vi "hold_queues_in_memory.vi"   [LabVIEW 2013]
uses:
  global variables.vi
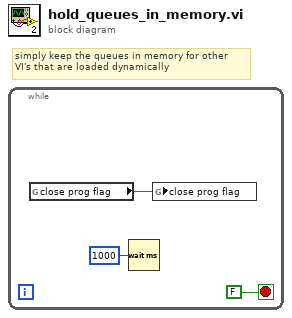
[diagram p0: block diagram]
diagram:
  # "simply keep the queues in memory for other\nVI's that are loaded dynamically"
  n1 = while {
    stop <- FALSE stop-if-true
    n2 = global read "global variables.vi" "close prog flag"() -> (w1:bool)
    n3 = Wait (ms)(milliseconds to wait=u32 1000) -> ()  [unwired: 1 out]
    n4 = global write "global variables.vi" "close prog flag"(w1) -> ()
  }
